vi "Heat2D_X Apply BC.vi"(6 "F(n+1)+F(n)":dbl[][](array[numeric]), 8 "Extended U(n)":dbl[][](array[numeric]), 9 "Coefficients":T1, 10 "step":i32, 11 "Boundary Condition":cluster{"type":T2, "Value":dbl[][]}[](array[cluster]) {"type" items=["Dirichlet", "Neumann"]}) -> (2 "U Right":dbl[](array[numeric]), 3 "U Left":dbl[](array[numeric]))   [LabVIEW 2020, in "NI_PDE.lvlib"]
uses:
  <vilib>/gmath/NI_PDE.lvlib
  <vilib>/gmath/pde.llb/Common/PDE_BC Type.ctl
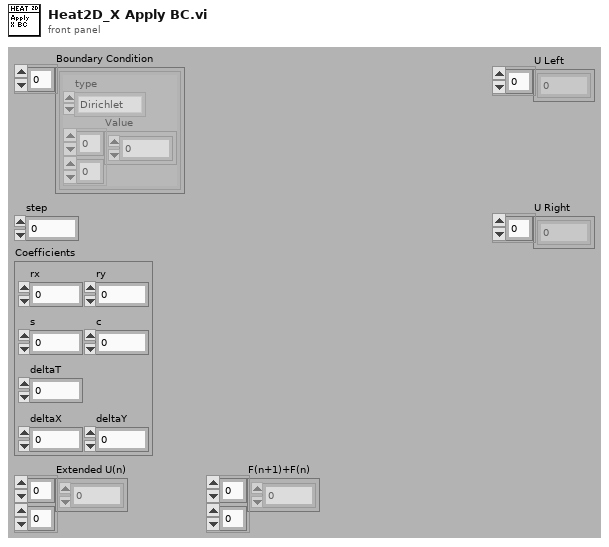
[diagram p1: front panel]
types:
  T1 = cluster{"rx":dbl, "ry":dbl, "s":dbl, "c":dbl, "deltaT":dbl, "deltaX":dbl, "deltaY":dbl}
  T2 = typedef "NI_PDE.lvlib/PDE_BC Type.ctl" = i32
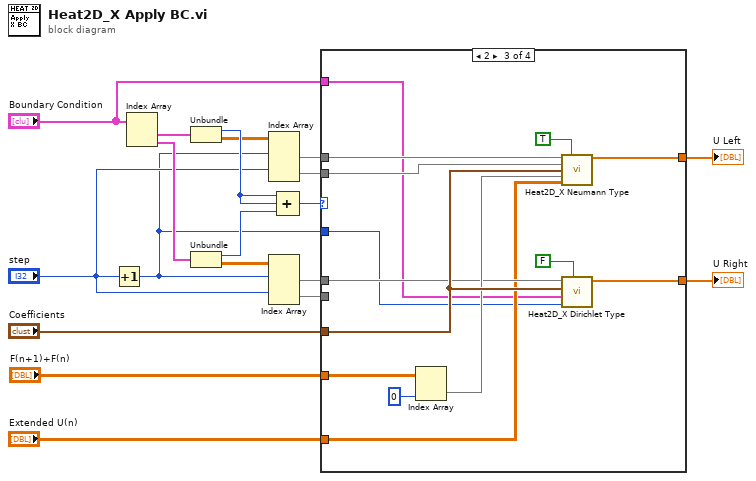
[diagram p0: block diagram]
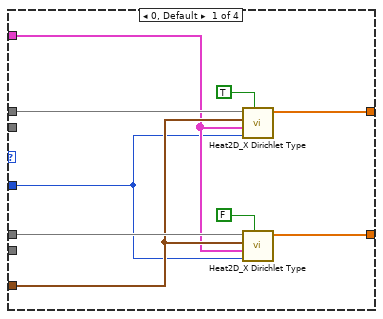
[diagram p2: hidden frame]
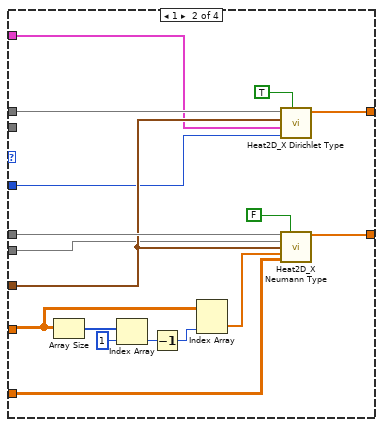
[diagram p3: hidden frame]
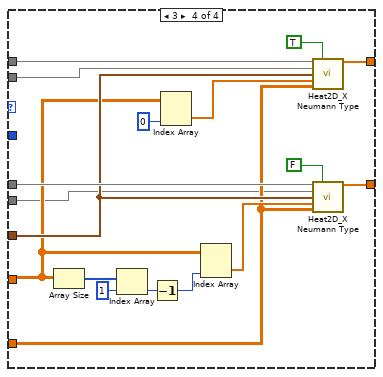
[diagram p4: hidden frame]
diagram:
  n1 = Increment(x="step") -> (x+1=w1:i32)
  n2 = Index Array(array="Boundary Condition") -> (element #1=w11:cluster{"type":T2, "Value":dbl[][]}, element #2=w12:cluster{"type":T2, "Value":dbl[][]})  [unwired: 2 in]
  n3 = Unbundle(w11) -> ("type"=w15:T2, "Value"=w13:dbl[][])
  n4 = Unbundle(w12) -> ("type"=w16:T2, "Value"=w14:dbl[][])
  n5 = Index Array(array=w13, index (row) #1=w1, index (row) #2="step") -> (element #1=w18:dbl[], element #2=w5:dbl[])  [unwired: 2 in]
  n6 = Index Array(array=w14, index (row) #1=w1, index (row) #2="step") -> (element #1=w19:dbl[], element #2=w3:dbl[])  [unwired: 2 in]
  n7 = Compound Arithmetic op=ADD(w15, w15, w16) -> (w17:T2)
  n8 = case shown="2" w17 {
    tunnel: w18 -> [w26 w44 w58 w70]
    tunnel: w19 -> [w27 w43 w54 w77]
    tunnel: [w25 w45 w57 w71] -> w7
    tunnel: [w28 w41 w53 w76] -> w6
    tunnel: "F(n+1)+F(n)" -> [_ w37 w55 w68]
    tunnel: "Extended U(n)" -> [_ w35 w52 w66]
    tunnel: "Coefficients" -> [w24 w42 w59 w69]
    tunnel: w5 -> [_ _ w50 w63]
    tunnel: w3 -> [_ w33 _ w62]
    tunnel: "Boundary Condition" -> [w21 w30 w48 _]
    tunnel: w1 -> [w20 w29 w46 _]
    frame 0, Default {
      n9 = call <vilib>:"Heat2D_X Dirichlet Type.vi"("Left?"=TRUE, "step (n+1)"=w20, "Boundary Condition"=w21, "Coefficients"=w24, "BC Value"=w26) -> ("U"=w25:dbl[])  [unwired: 6 out]
      n10 = call <vilib>:"Heat2D_X Dirichlet Type.vi"("Left?"=FALSE, "step (n+1)"=w20, "Boundary Condition"=w21, "Coefficients"=w24, "BC Value"=w27) -> ("U"=w28:dbl[])  [unwired: 6 out]
    }
    frame 1 {
      n11 = Array Size(array=w37) -> (size(s)=w40:i32[])
      n12 = Index Array(array=w40, index=1) -> (element=w38:i32)
      n13 = Decrement(x=w38) -> (x-1=w32:i32)
      n14 = Index Array(array=w37, index (col)=w32) -> (element=w36:dbl[])  [unwired: 1 in]
      n15 = call <vilib>:"Heat2D_X Dirichlet Type.vi"("Left?"=TRUE, "step (n+1)"=w29, "Boundary Condition"=w30, "Coefficients"=w42, "BC Value"=w44) -> ("U"=w45:dbl[])  [unwired: 6 out]
      n16 = call <vilib>:"Heat2D_X Neumann Type.vi"("BC Value(n+1)"=w43, "Left?"=FALSE, "BC Value(n)"=w33, "Coefficients"=w42, "F(n+1)+F(n)"=w36, "Extended U(n)"=w35) -> ("RHS"=w41:dbl[])  [unwired: 9 out]
    }
    frame 2 {
      n17 = Index Array(array=w55, index (col)=0 ("disabled index (col)")) -> (element=w56:dbl[])  [unwired: 1 in]
      n18 = call <vilib>:"Heat2D_X Neumann Type.vi"("BC Value(n+1)"=w58, "Left?"=TRUE, "BC Value(n)"=w50, "Coefficients"=w59, "F(n+1)+F(n)"=w56, "Extended U(n)"=w52) -> ("RHS"=w57:dbl[])  [unwired: 9 out]
      n19 = call <vilib>:"Heat2D_X Dirichlet Type.vi"("Left?"=FALSE, "step (n+1)"=w46, "Boundary Condition"=w48, "Coefficients"=w59, "BC Value"=w54) -> ("U"=w53:dbl[])  [unwired: 6 out]
    }
    frame 3 {
      n20 = Array Size(array=w68) -> (size(s)=w75:i32[])
      n21 = Index Array(array=w75, index=1) -> (element=w73:i32)
      n22 = Decrement(x=w73) -> (x-1=w61:i32)
      n23 = Index Array(array=w68, index (col)=0 ("disabled index (col)")) -> (element=w67:dbl[])  [unwired: 1 in]
      n24 = Index Array(array=w68, index (col)=w61) -> (element=w72:dbl[])  [unwired: 1 in]
      n25 = call <vilib>:"Heat2D_X Neumann Type.vi"("BC Value(n+1)"=w70, "Left?"=TRUE, "BC Value(n)"=w63, "Coefficients"=w69, "F(n+1)+F(n)"=w67, "Extended U(n)"=w66) -> ("RHS"=w71:dbl[])  [unwired: 9 out]
      n26 = call <vilib>:"Heat2D_X Neumann Type.vi"("BC Value(n+1)"=w77, "Left?"=FALSE, "BC Value(n)"=w62, "Coefficients"=w69, "F(n+1)+F(n)"=w72, "Extended U(n)"=w66) -> ("RHS"=w76:dbl[])  [unwired: 9 out]
    }
  }
  "U Left" <- w7
  "U Right" <- w6
